vi "adam-thermocouple-input.vi"(0 "VISA Refnum in":refnum<visa-resource-name>, 1 "Chassis Settings":T2, 9 "chassis-slot":i32, 11 "error in (no error)":errorcluster, 12 "last cmd in":string, 13 "last read buffer":string) -> (4 "VISA Refnum out":refnum<visa-resource-name>, 6 "Thermocouple Inputs (degC)":T1, 8 "cmd out":string, 10 "read-buffer out":string, 14 "cmd aknowledged":bool, 15 "error out":errorcluster)   [LabVIEW 2024]
uses:
  controls/adam-5000-serial-settings.ctl
  controls/thermocouple-input-cluster.ctl
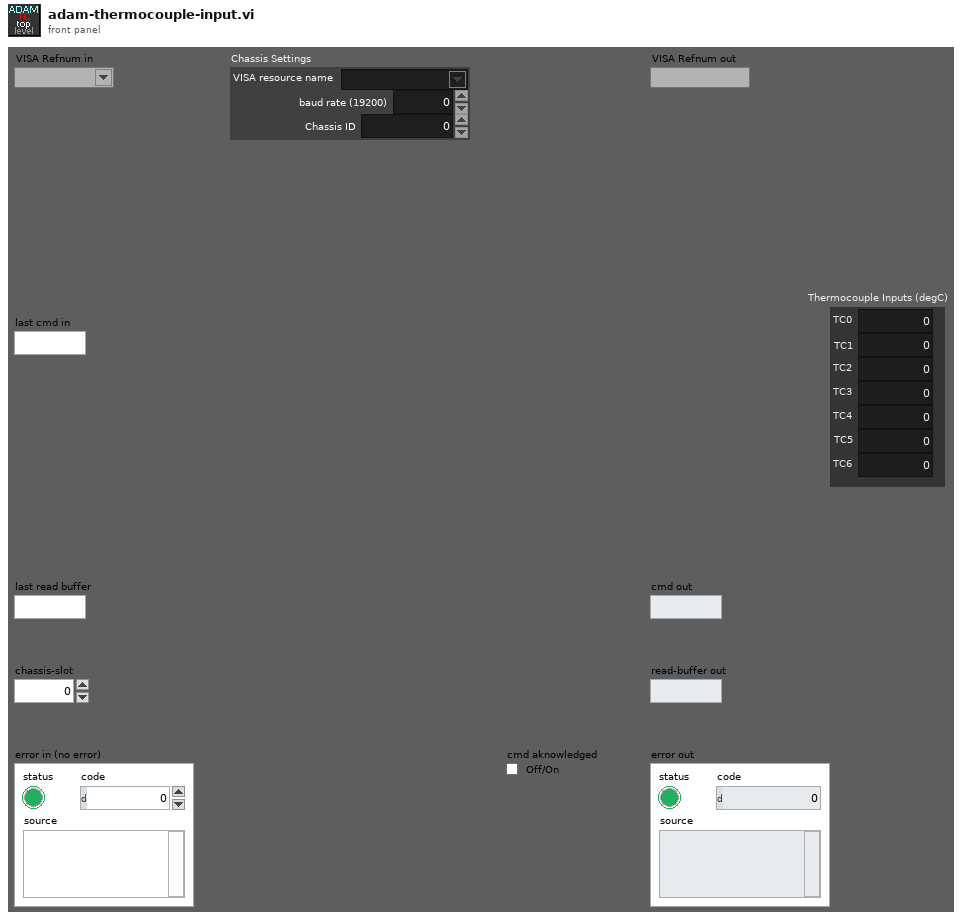
[diagram p1: front panel]
types:
  T1 = typedef "thermocouple-input-cluster.ctl" = cluster{"TC0":dbl, "TC1":dbl, "TC2":dbl, "TC3":dbl, "TC4":dbl, "TC5":dbl, "TC6":dbl}
  T2 = typedef "adam-5000-serial-settings.ctl" = cluster{"VISA resource name":refnum<visa-resource-name>, "baud rate (19200)":u32, "Chassis ID":u8}
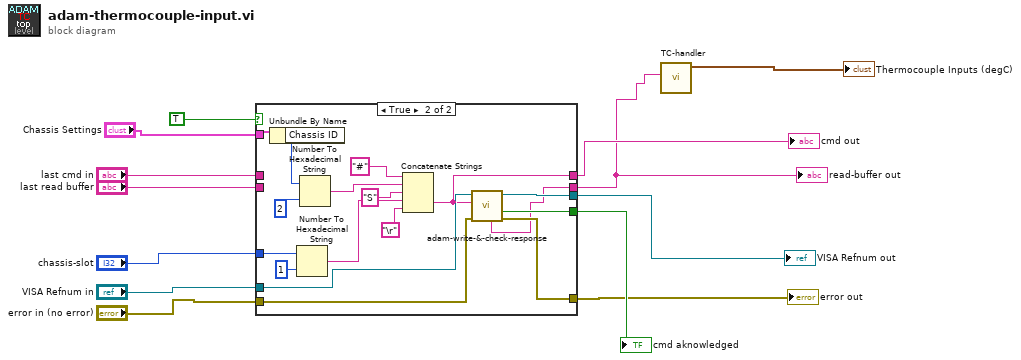
[diagram p0: block diagram]
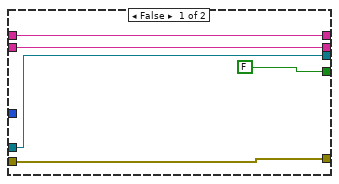
[diagram p2: hidden frame]
diagram:
  n1 = case shown="True" TRUE {
    tunnel: "VISA Refnum in" -> [w18 w31]
    tunnel: "error in (no error)" -> [w16 w30]
    tunnel: [w16 w29] -> w6
    tunnel: [w18 w28] -> w7
    tunnel: [FALSE ("cmd aknowledged") w27] -> w13
    tunnel: [w15 w19] -> w2
    tunnel: [w14 w26] -> w12
    tunnel: "Chassis Settings" -> [_ w24]
    tunnel: "chassis-slot" -> [_ w23]
    tunnel: "last read buffer" -> [w15 _]
    tunnel: "last cmd in" -> [w14 _]
    frame False {
    }
    frame True {
      n2 = Unbundle By Name(w24) -> ("Chassis ID"=w35:u8)
      n3 = Number To Hexadecimal String(1:i16 1 ("width (-)"), 2:w23) -> (0:w21:string)
      n4 = Number To Hexadecimal String(1:i16 2 ("width (-)"), 2:w35) -> (0:w33:string)
      n5 = Concatenate Strings("#" ("string"), w33, "S" ("string"), w21, "\r") -> (w26:string)
      n6 = call "adam-write-&-check-response.vi"("error in (no error)"=w30, "write buffer"=w26, "VISA resource name"=w31) -> ("error out"=w29:errorcluster, "cmd aknowledged"=w27:bool, "VISA resource name out"=w28:refnum<visa-resource-name>, "read buffer"=w19:string)  [unwired: 3 in, 2 out]
    }
  }
  "cmd aknowledged" <- w13
  "cmd out" <- w12
  "read-buffer out" <- w2
  "VISA Refnum out" <- w7
  "error out" <- w6
  n7 = call "TC-handler.vi"("read buffer in"=w2) -> ("Thermocouple Inputs (degC)"=→"Thermocouple Inputs (degC)":T1)  [unwired: 10 in]
